vi "Magnet_PS_Main.vi"(10 "Comms Layer":T3, 11 "VISA iPS":refnum<visa-resource-name>="COM6" caption="VISA") -> (3 "Output Current (A)":dbl format="%.2g")   [LabVIEW 2019]
uses:
  Mercury iXX Modules/Public/Controls/Comms Transport Layer.ctl
  Mercury iXX Modules/Public/Libraries/Magnet/Controls/PSU Actions.ctl
  <vilib>/Instr/_visa.llb/VISA Flush IO Buffer Mask.ctl
  Magnet_PS_Global.vi
  Mercury iXX Modules/Public/Libraries/Magnet/Configuration/Set/PSU Action Status (Set).vi
  Mercury iXX Modules/Public/Libraries/Magnet/Signals/Set/Target Current (Set).vi
  Mercury iXX Modules/Mercury iXX.lvlib
  Mercury iXX Modules/Public/Libraries/Magnet.lvlib
panel:
  in  "recon_ami1700":bool
  out "lock_time_now":i32 caption="Time Elapsed"
  in  "lock_time_max":i32=600 caption="Max Time"
  in  "enable_time_limit":bool=TRUE caption="Time Limit"
  out "High BG Light?":bool
  out "current_diff":u32(colorbox) caption="Current Difference Status"
  in  "lock_unusual_manip":bool=TRUE caption="Unusual Controls"
  out "quenched_light":bool caption="Quenched"
  out "PSU_stat_hex":i32 caption="Status" format="%x"
  out "PSU_Stat":T1 caption="PSU Status"
  out "clamped_light":bool caption="Clamped"
  out "pd read":string
  out "pd_shim_2":bool
  out "pd_shim_1":bool
  in  "termination char\n(0xA = '\\n' = LF)":u8=10 format="%.0x"
  in  "VISA_ps_pd":refnum<visa-resource-name>="COM40"
  out "Status":bool
  in  "ps_ip_addr":string="192.168.24.91" caption="IP Addr."
  in  "LHe_probe_int_samp":i8=5 caption="Interval (min)"
  in  "LHe_probe_mode":enum16{"CONT", "HOLD"}(ring) caption="LHe Mode"
  in  "curr_preset":T2(ring) caption="Presets"
  in  "relay_port":u16=6722 caption="Port"
  in  "relay_address":string="192.168.24.184" caption="Addr."
  out "He Liter":dbl(slide) caption="Calibrated" scale=0.0..145.0
  out "Last Update":timestamp format="%<%Y-%m-%d %H:%M:%S>T"
  out "iPS_msg":string caption="Msg."
  out "AMI1700_status":bool caption="Status"
  in  "AMI1700_port":u16=7180 caption="Port"
  in  "AMI1700_address":string="192.168.24.134" caption="Addr."
  in  "stop":bool
  out "shim_relay_message":string caption="Msg."
  out "shim_relay_status":bool caption="Status"
  in  "Shim 2":bool caption="#2"
  in  "Shim 1":bool caption="Shim Switch Heater #1"
  in  "Save Button":bool
  in  "x":dbl=14.889566783098592 format="%#_13g"
  in  "Current NMR Central Frequency:":dbl
  in  "y":dbl=20.0
  out "SAFETY TIMEOUT":u8(slide) scale=0.0..60.0
  in  "safemode":bool
  out "Timer":dbl
  in  "Help Button":bool
  out "help_msg":string="To ramp the current above 74.8 A, or faster than 2 A/min (for I<40A), 1 A/min (for 40A<I<63A) or 0.5 A/min (for I>63A), please enter the correct password.\n\nBaseline Mode: Toggle on to ramp the magnet to 1 A below the set point for the purposes of taking a baseline. Toggle off to ramp back to the set point. If the switch heater is off, it will be turned on when this button is pressed.\n\nSafety Mode: While toggled on, switch heater will automatically turn off after 20 minutes of inactivity. Enter password to change timeout duration."
  in  "Special Functions":bool
  out "Baselinetext":string
  in  "Target Species:":dbl(ring)=42.576 items=["Proton"=42.576, "Deuteron"=6.536]
  out "Heater Status 2":u8(slide) scale=0.0..60.0
  in  "Baseline Mode":bool
  out "Heater Status":u8(slide) scale=0.0..60.0
  out "big_message":string
  in  "Set Target Frequency (MHz):":dbl max=213.8870019787944
  in  "Set Target Field (T):":dbl max=5.02365186909983 format="%#_5g"
  in  "Axis Group":string(combo)="GRPZ"
  in  "Target Current":dbl max=74.8 format="%#_5g"
  out "N2 Level":dbl(slide) scale=0.0..100.0
  out "He Level":dbl(slide) scale=0.0..45.0
  in  "all_cont_lock":bool caption="All Controls"
  out "Zerolight":bool
  out "Setlight":bool
  out "Holdlight":bool
  out "Persistent Current (A)":dbl format="%.2g"
  in  "PASSWORD:":string
  out "Heater Indicator 3":bool caption="Main Switch Heater"
  in  "Switch Heater":bool caption="Toggle"
  in  "Ramp Rate (A/min)":dbl=0.5 min=0.0 max=2.0 format="%_2f"
  out "Set Target Current (A):":cluster{dbl, dbl}(knob)={0.0, 68.56622626412835} scale=0.0..120.0 scale format="%#_5g"
  in  "To Zero":bool
  in  "To Set":bool
  in  "Hold":bool
  out "Waveform Chart":cluster{"[0]":dbl, "[1]":dbl}(graph)
  out "Output Voltage (V)":dbl format="%.3g"
  out "iPS_status":bool caption="Status"
  out "String 2":string
  # "Magnet Power Supply"
  # "/"
  # "s"
  # "For Drift Calibration:"
  # "Mercury iPS"
  # "%"
  # "L"
  # "%"
  # "Shim Relay"
  # "Known as bad."
  # "AMI1700"
  # "The ramp rate is auto-lowered when exceeding the limit that is defined in hardware as a function of output current."
  # "This toggle button changes the main & shim switch heaters together."
  # "PD Reading"
  # "Photodiodes"
  # "(hex)"
  # "Unusual Controls:\n* Press \"To Set\" or \"To Zero\" when the main+shim heaters are not all ON or OFF.\n* Change the heater status when the PS is not in \"Hold\".\n* Change the heater status when Output current != Presistent Current.\nYou might hover the mouse cursor on the \"Unusual Controls\" button\nto find the reason why controls are prohibited."
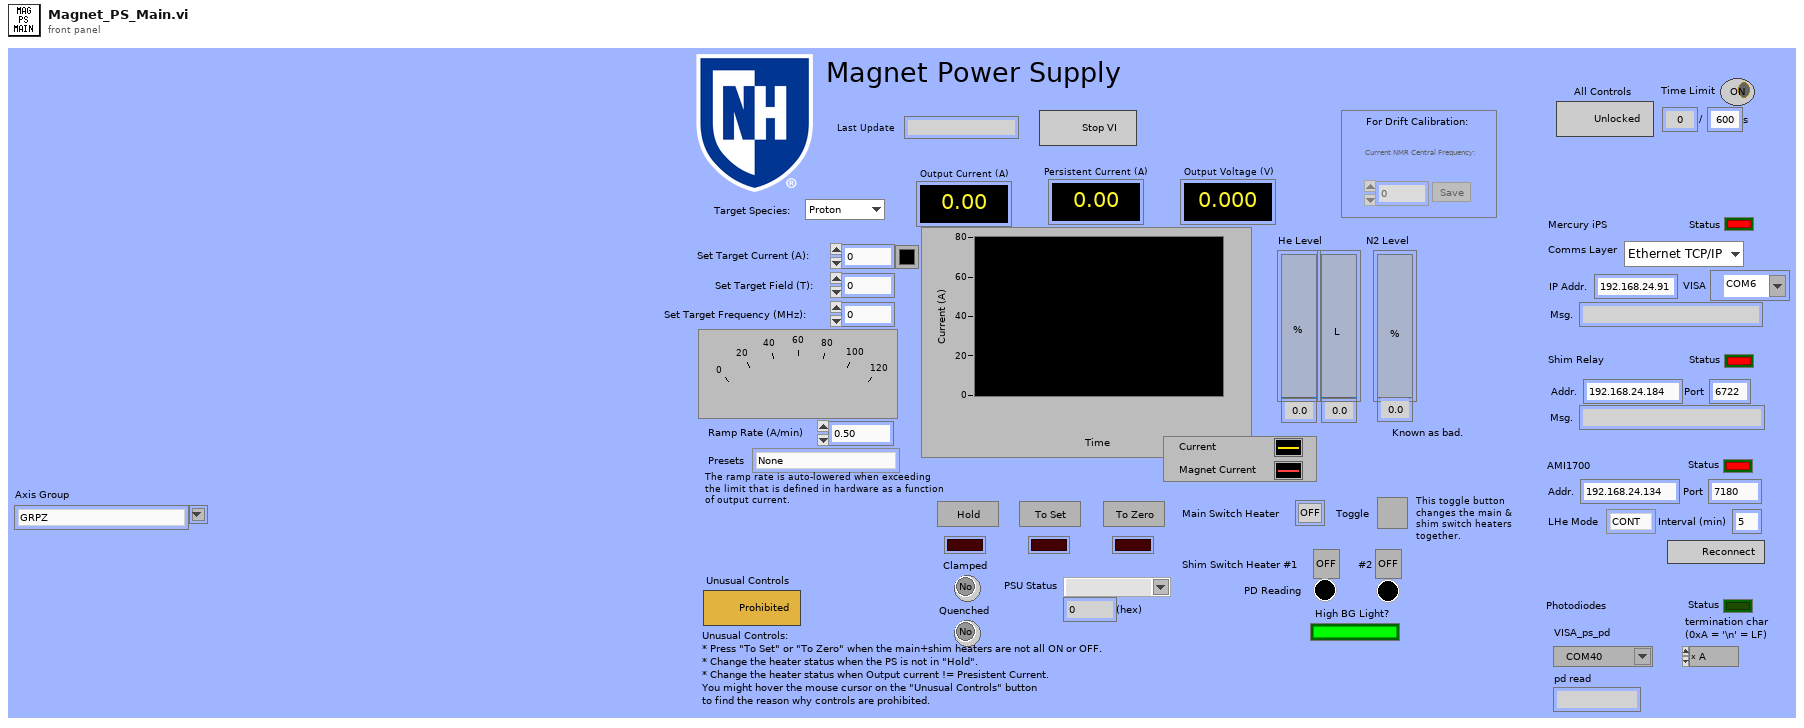
[diagram p1: front panel]
types:
  T1 = typedef "Mercury iXX.lvlib/Magnet.lvlib/PSU Actions.ctl" = string
  T2 = enum16{"None", "Up to 45 A at 2 A/m", "Up to 63 A at 1 A/m", "Up to 74.51 A at 0.5 A/m", "Up to 74.47 A at 0.5 A/m", "Down to 74 A at 0.5 A/m", "Down to 63 A at 0.5 A/m", "Down to 45 A at 1 A/m", "Down to 0 A at 2 A/m", "Down to 0 A at 0.5 A/m"}
  T3 = typedef "Mercury iXX.lvlib/Comms Transport Layer.ctl" = enum16{"Ethernet TCP/IP", "USB", "ISOBus - RS-232", "GPIB"}
  T4 = typedef "VISA Flush IO Buffer Mask.ctl" = u16
  T5 = typedef "Mercury iXX.lvlib/ISOBus Address.ctl" = i32
  T6 = typedef "Mercury iXX.lvlib/Mercury Reference.ctl" = cluster{"Comms":refnum<visa-resource-name>, "Device ID":string[], "Comms Layer":T3, "Command":string, "Query reference":T7}
  T7 = typedef "Mercury iXX.lvlib/Query Dynamic Reference.ctl" = refnum<vi>
  T8 = enum8{"Enabled", "Disabled", "Disabled and Grayed Out"}
  T9 = enum16{"None", "Up: 45 A, 2 A/m", "Up: 63 A, 1 A/m", "Up: 74.78 A, 0.5 A/m", "Down: 63 A, 0.5 A/m", "Down: 45 A, 1 A/m", "Down: 0 A, 2 A/m"}
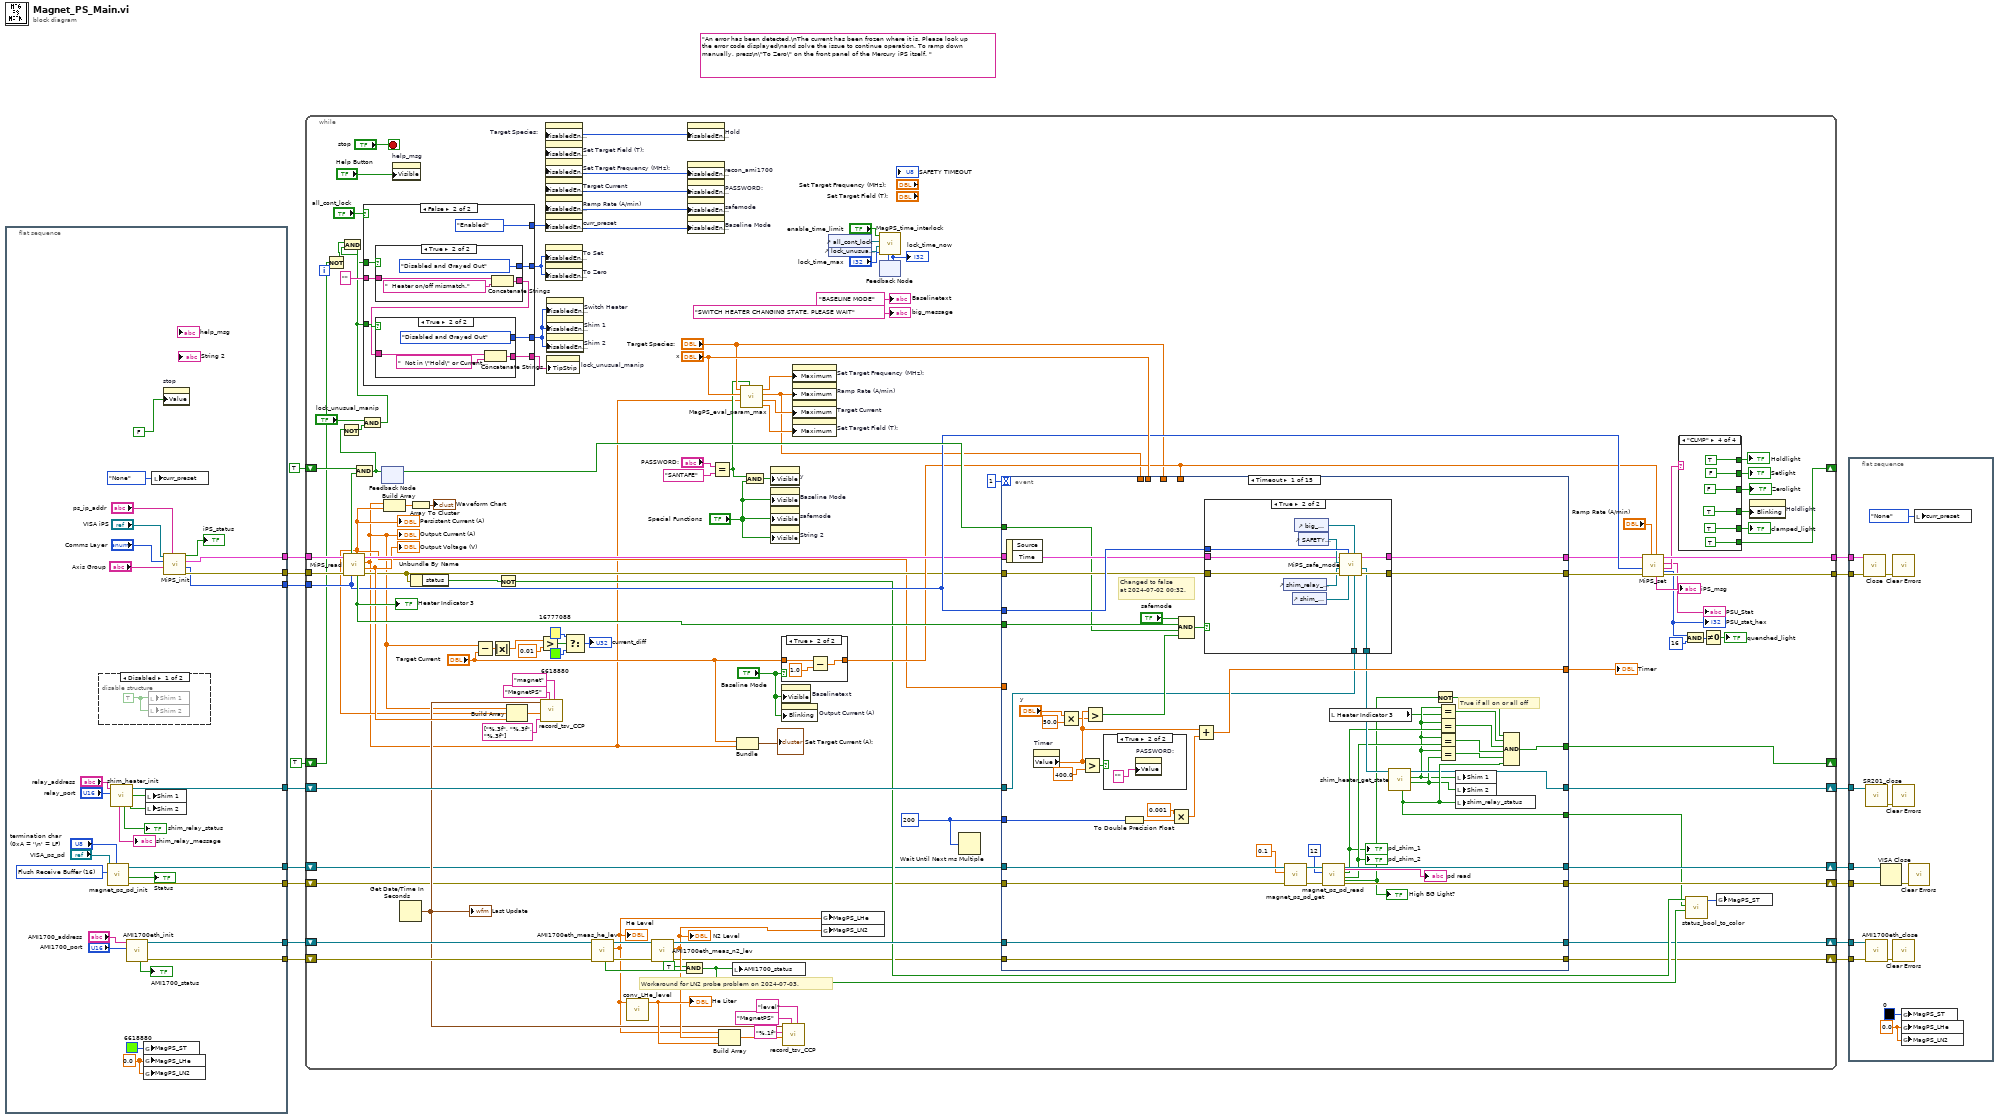
[diagram p0: block diagram]
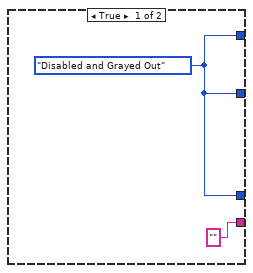
[diagram p3: hidden frame]
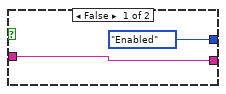
[diagram p4: hidden frame]
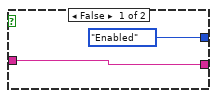
[diagram p5: hidden frame]
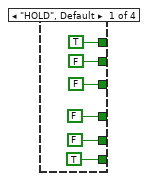
[diagram p7: hidden frame]
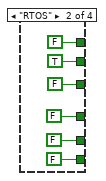
[diagram p8: hidden frame]
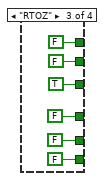
[diagram p9: hidden frame]
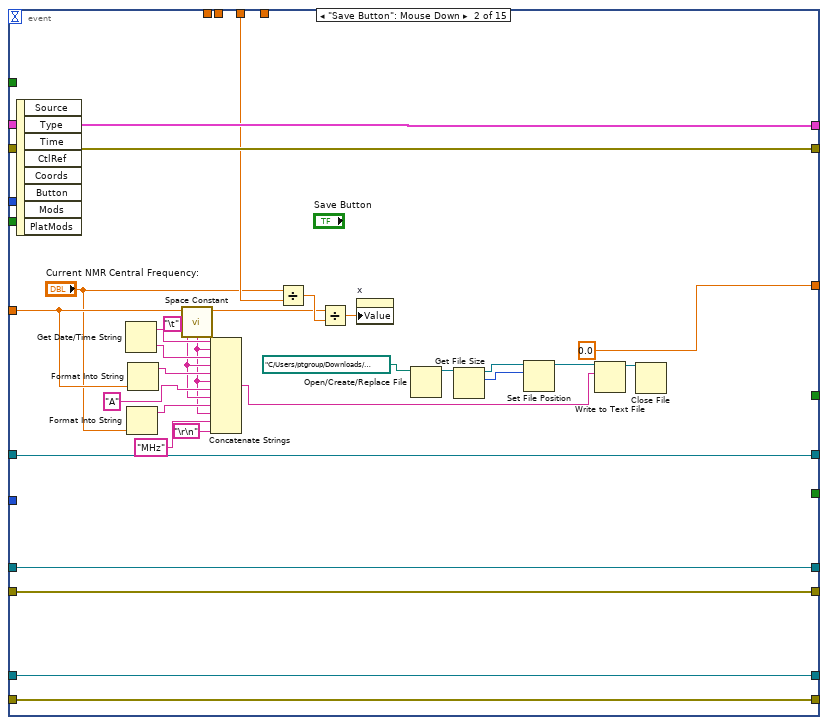
[diagram p12: hidden frame]
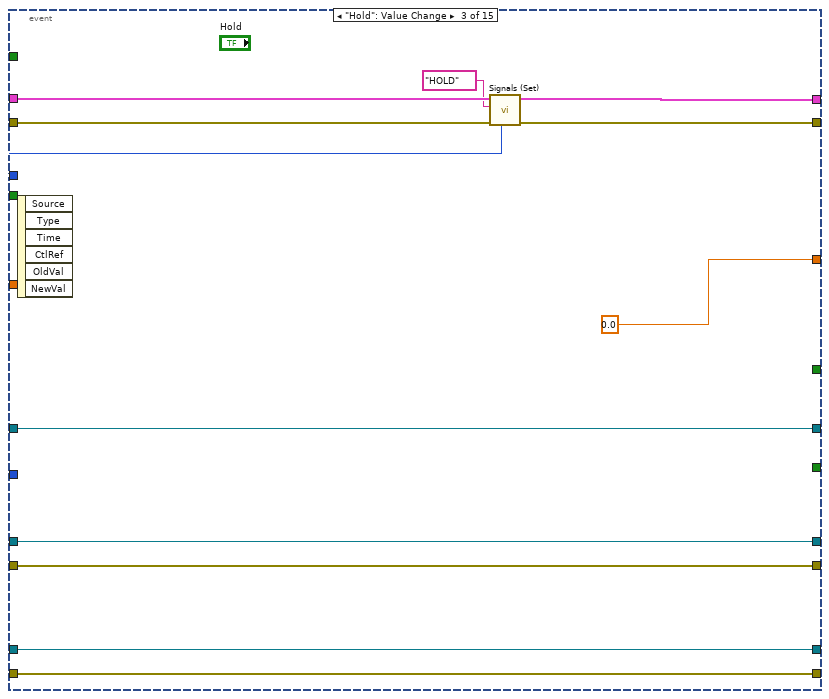
[diagram p13: hidden frame]
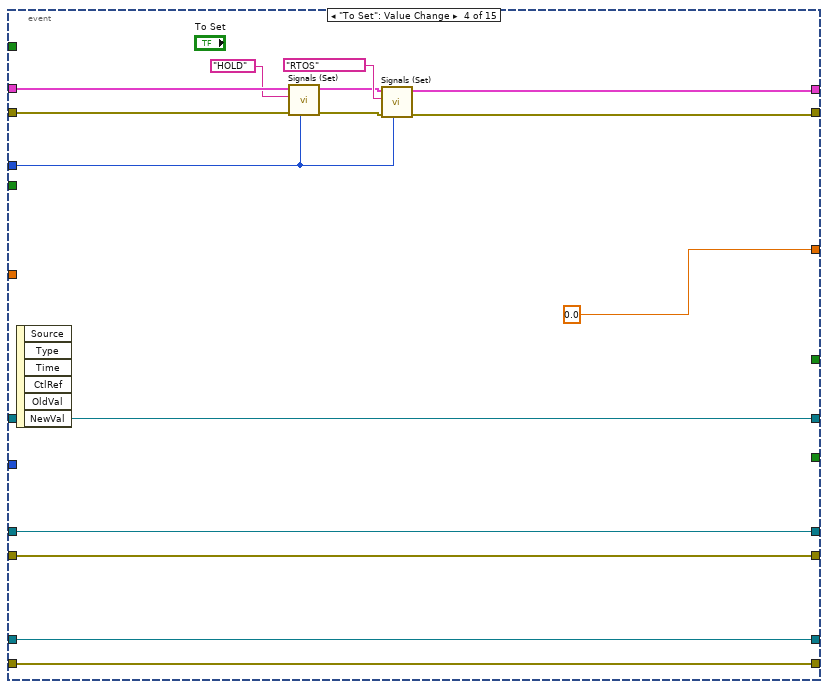
[diagram p14: hidden frame]
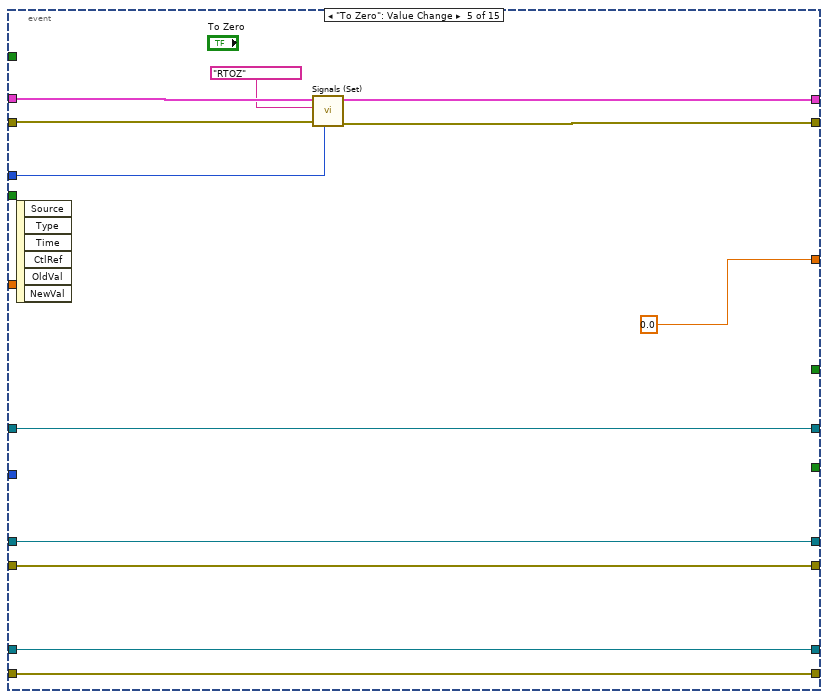
[diagram p15: hidden frame]
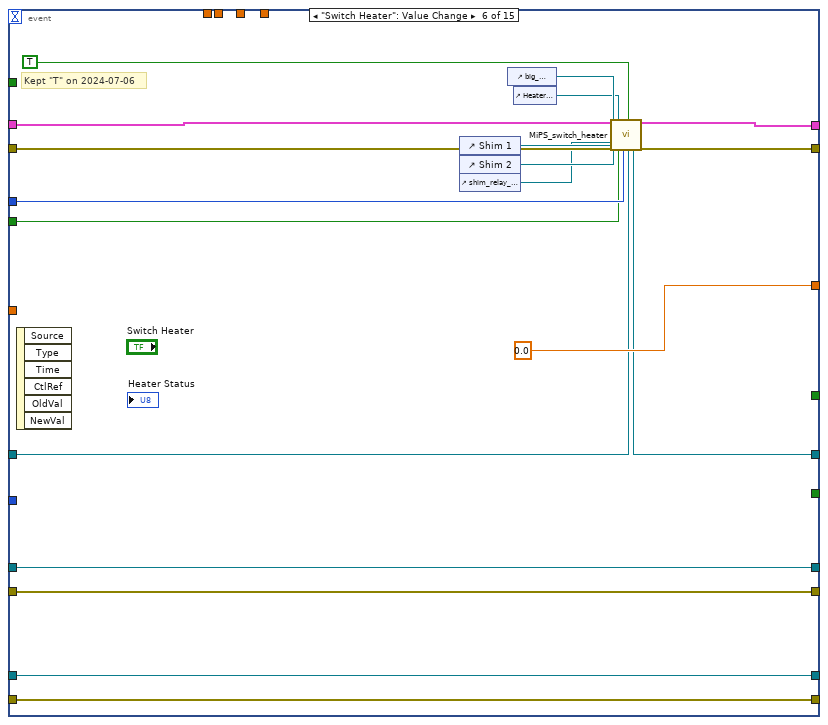
[diagram p16: hidden frame]
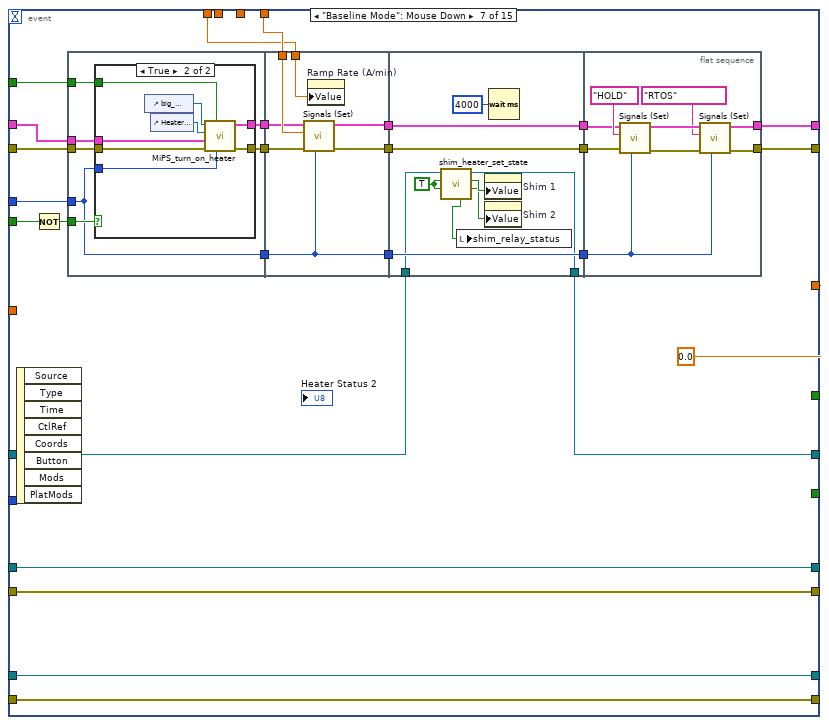
[diagram p17: hidden frame]
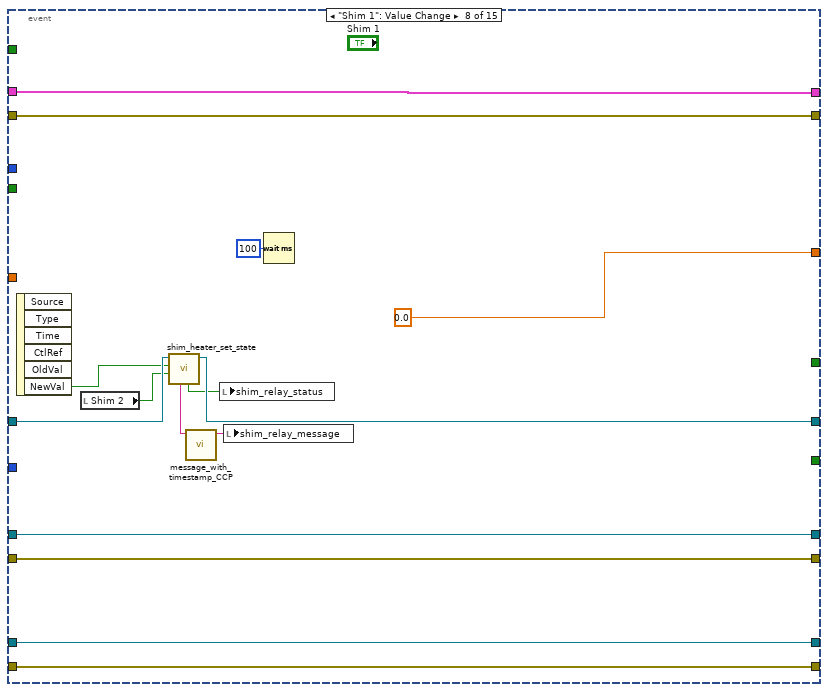
[diagram p19: hidden frame]
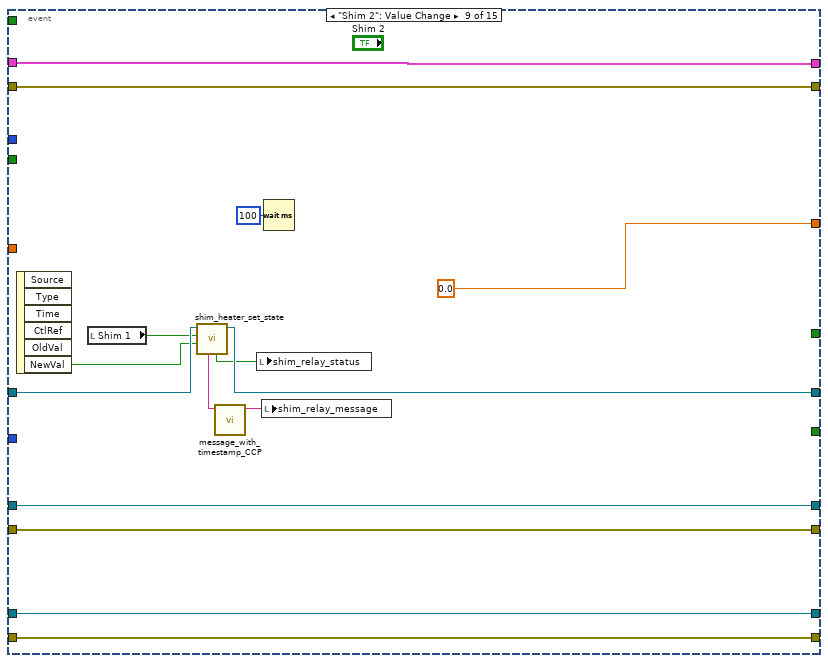
[diagram p20: hidden frame]
diagram:
  (unwired) "An error has been detected.\nThe current has been frozen where it is. Please look up the error code displayed\nand solve the issue to continue operation. To ramp down manually, press\n\"To Zero\" on the front panel of the Mercury iPS itself. " ("message")
  n1 = flat-sequence {
    tunnel: [w46] -> w17
    tunnel: [w45] -> w16
    tunnel: [w42] -> w13
    tunnel: [w37] -> w12
    tunnel: [w36] -> w11
    tunnel: [w32] -> w7
    tunnel: [w19] -> w3
    tunnel: [w21] -> w5
    frame #0 {
      w23 = T4 16 items=["Flush Receive Buffer"=16, "Write Transmit Buffer to Device"=32, "Flush Receive Buffer (No I/O)"=64, "Flush Transmit Buffer"=128] ("Mask")
      w26 = 0.0 ("MagPS_LHe")
      n2 = disable-structure shown="Disabled" {
        frame Disabled {
          w48 = TRUE ("Shim 1")
          n3 = local write "Shim 1"(w48) -> ()
          n4 = local write "Shim 2"(w48) -> ()
        }
        frame Enabled {
        }
      }
      n5 = call "magnet_ps_pd_init.vi"("termination char\n(0xA = '\\n' = LF)"="termination char\n(0xA = '\\n' = LF)", "Mask"=w23, "VISA resource name"="VISA_ps_pd") -> ("error out"=w19:errorcluster, "Status"=→"Status":bool, "VISA resource name out"=w21:refnum<visa-resource-name>)  [unwired: 6 in]
      n6 = call "shim_heater_init.vi"("port"="relay_port", "address"="relay_address") -> ("ch2"=w28:bool, "ch1"=w29:bool, "conn_id"=w32:refnum<k5>, "status"=→"shim_relay_status":bool, "message"=→"shim_relay_message":string)  [unwired: 4 in, 1 out]
      n7 = call "AMI1700eth_init.vi"("port"="AMI1700_port", "address"="AMI1700_address") -> ("error out"=w36:errorcluster, "conn_id"=w37:refnum<k5>, "status"=→"AMI1700_status":bool)  [unwired: 7 in]
      n8 = global write "Magnet_PS_Global.vi" "MagPS_ST"(u32 6618880 ("MagPS_ST")) -> ()
      n9 = global write "Magnet_PS_Global.vi" "MagPS_LHe"(w26) -> ()
      n10 = global write "Magnet_PS_Global.vi" "MagPS_LN2"(w26) -> ()
      n11 = local write "Shim 1"(w29) -> ()
      n12 = local write "Shim 2"(w28) -> ()
      n13 = local write "curr_preset"(T2."None" ("curr_preset")) -> ()
      n14 = property on="stop" class="Bool (strict)"("Value"=FALSE ("stop")) -> ()  [unwired: 2 in, 2 out]
      n15 = call "MiPS_init.vi"("ip_addr"="ps_ip_addr", "Axis Group"="Axis Group", "Comms Layer"="Comms Layer", "VISA in"="VISA iPS") -> ("error out"=w45:errorcluster, "ISOBUS address"=w42:T5, "ref_out"=w46:T6, "status"=→"iPS_status":bool)  [unwired: 4 in]
    }
  }
  n16 = while {
    tunnel: w17 -> [w156]
    tunnel: w16 -> [w157]
    tunnel: [w150] -> w15
    tunnel: [w149] -> w14
    tunnel: w13 -> [w129]
    shift-right: [w54] -> w10
    shift-left: w12 -> [w132]
    shift-right: [w55] -> w9
    shift-left: w11 -> [w134]
    shift-right: [w118] -> _
    shift-left: TRUE -> [w117]
    shift-right: [w74] -> w6
    shift-left: w7 -> [w105]
    shift-right: [w94] -> w4
    shift-left: w5 -> [w95]
    shift-right: [w92] -> w2
    shift-left: w3 -> [w93]
    shift-right: [w73] -> _
    shift-left: TRUE -> [w76]
    stop <- "stop" stop-if-true
    w137 = u32 200 ("millisecond multiple")
    # "Workaround for LN2 probe problem on 2024-07-03."
    n17 = Not(x=w76) -> (.not. x?=w50:bool)
    n18 = call "MiPS_read.vi"("ISOBUS address"=w129, "error in"=w157, "ref_in"=w156) -> ("error out"=w107:errorcluster, "Voltage"=w108:dbl, "Current"=w71:dbl, "ref_out"=w128:T6, "heater_status"=w151:bool, "Persistant Current"=w85:dbl, "current_in_range"=w127:bool)  [unwired: 2 in]
    "Output Current (A)" <- w71
    "Output Voltage (V)" <- w108
    "Heater Indicator 3" <- w151
    "Persistent Current (A)" <- w85
    n19 = And(x=w117, y=w127) -> (x .and. y?=w81:bool)
    n20 = Not(x=w81) -> (.not. x?=w82:bool)
    n21 = And(x="lock_unusual_manip", y=w82) -> (x .and. y?=w52:bool)
    n22 = And(x=w50, y=w52) -> (x .and. y?=w51:bool)
    n23 = case shown="False" "all_cont_lock" {
      tunnel: [w164 w172] -> w83
      tunnel: w52 -> [_ w167]
      tunnel: [w164 T8."Enabled" ("Disabled")] -> w53
      tunnel: [w164 w170] -> w80
      tunnel: ["" ("f") w169] -> w79
      tunnel: "" ("f") -> [_ w168]
      tunnel: w51 -> [_ w165]
      frame True {
        w164 = T8."Disabled and Grayed Out" ("Disabled")
      }
      frame False {
        n24 = case shown="True" w165 {
          tunnel: [T8."Enabled" ("Disabled") T8."Disabled and Grayed Out" ("Disabled")] -> w170
          tunnel: w168 -> [w173 w177]
          tunnel: [w173 w176] -> w166
          frame False {
          }
          frame True {
            n25 = Concatenate Strings(w177, "  Heater on/off mismatch." ("string")) -> (w176:string)
          }
        }
        n26 = case shown="True" w167 {
          tunnel: [T8."Enabled" ("Disabled") T8."Disabled and Grayed Out" ("Disabled")] -> w172
          tunnel: [w179 w183] -> w169
          tunnel: w166 -> [w179 w182]
          frame False {
          }
          frame True {
            n27 = Concatenate Strings(w182, "  Not in \"Hold\" or Current mismatch." ("msg_heater_manip")) -> (w183:string)
          }
        }
      }
    }
    n28 = feedback-in #1(w81) -> ()
    n29 = feedback #1() -> (w144:bool)  [unwired: 1 in]
    n30 = Build Array(w71, w85) -> (w148:dbl[])
    n31 = property on="help_msg" class="Str"("Visible"="Help Button") -> ()  [unwired: 2 in, 2 out]
    n32 = Get Date/Time In Seconds() -> (seconds since 1Jan1904=w98:timestamp)
    "Last Update" <- w98
    n33 = Array To Cluster(array=w148) -> (cluster=→"Waveform Chart":cluster{"[0]":dbl, "[1]":dbl})
    n34 = Unbundle By Name(w107) -> ("status"=w106:bool)
    n35 = Subtract(x=w71, y="Target Current") -> (x-y=w70:dbl)
    n36 = Absolute Value(x=w70) -> (abs(x)=w68:dbl)
    n37 = Not(x=w106) -> (.not. x?=w103:bool)
    n38 = Build Array(w71, w85, w108) -> (w110:dbl[])
    n39 = Greater?(x=w68, y=0.01) -> (0:w67:bool)
    n40 = call "record_tsv_CCP.vi"("file_name"="magnet", "folder_name"="MagnetPS", "format_array"=string[] ["%.3f", "%.3f", "%.3f"], "value_array"=w110, "time"=w98) -> ()  [unwired: 5 in, 2 out]
    n41 = property on="Target Species:" class="Ring (strict)"("DisabledEnum"=w53) -> ()  [unwired: 2 in, 2 out]
    n42 = property on="Set Target Field (T):" class="DigNum (strict)"("DisabledEnum"=w53) -> ()  [unwired: 2 in, 2 out]
    n43 = property on="Set Target Frequency (MHz):" class="DigNum (strict)"("DisabledEnum"=w53) -> ()  [unwired: 2 in, 2 out]
    n44 = property on="Target Current" class="DigNum (strict)"("DisabledEnum"=w53) -> ()  [unwired: 2 in, 2 out]
    n45 = property on="Ramp Rate (A/min)" class="DigNum (strict)"("DisabledEnum"=w53) -> ()  [unwired: 2 in, 2 out]
    n46 = property on="curr_preset" class="Enum (strict)"("DisabledEnum"=w53) -> ()  [unwired: 2 in, 2 out]
    n47 = property on="To Set" class="Bool"("DisabledEnum"=w80) -> ()  [unwired: 2 in, 2 out]
    n48 = property on="To Zero" class="Bool"("DisabledEnum"=w80) -> ()  [unwired: 2 in, 2 out]
    n49 = property on="Switch Heater" class="Bool"("DisabledEnum"=w83) -> ()  [unwired: 2 in, 2 out]
    n50 = property on="Shim 1" class="Bool (strict)"("DisabledEnum"=w83) -> ()  [unwired: 2 in, 2 out]
    n51 = property on="Shim 2" class="Bool (strict)"("DisabledEnum"=w83) -> ()  [unwired: 2 in, 2 out]
    n52 = property on="lock_unusual_manip" class="Bool (strict)"("TipStrip"=w79) -> ()  [unwired: 2 in, 2 out]
    n53 = Select(t=u32 16777088 ("THCD401_ST"), s=w67, f=u32 6618880 ("THCD401_ST")) -> (s? t:f=→"current_diff":u32)
    n54 = call "AMI1700eth_meas_he_lev.vi"("error in"=w134, "conn_id_in"=w132) -> ("error out"=w133:errorcluster, "level"=w96:dbl, "conn_id_out"=w131:refnum<k5>, "status"=w130:bool)  [unwired: 5 in, 1 out]
    "He Level" <- w96
    n55 = call "conv_LHe_level.vi"("level_in"=w96) -> ("level_out"=w113:dbl)  [unwired: 10 in]
    "He Liter" <- w113
    n56 = call "AMI1700eth_meas_n2_lev.vi"("error in"=w133, "conn_id_in"=w131) -> ("error out"=w56:errorcluster, "level"=w100:dbl, "conn_id_out"=w104:refnum<k5>)  [unwired: 6 in, 1 out]
    "N2 Level" <- w100
    n57 = And(x=TRUE, y=w130) -> (x .and. y?=w101:bool)
    n58 = property on="Hold" class="Bool"("DisabledEnum"=w53) -> ()  [unwired: 2 in, 2 out]
    n59 = property on="recon_ami1700" class="Bool"("DisabledEnum"=w53) -> ()  [unwired: 2 in, 2 out]
    n60 = property on="PASSWORD:" class="Str"("DisabledEnum"=w53) -> ()  [unwired: 2 in, 2 out]
    n61 = property on="safemode" class="Bool (strict)"("DisabledEnum"=w53) -> ()  [unwired: 2 in, 2 out]
    n62 = property on="Baseline Mode" class="Bool (strict)"("DisabledEnum"=w53) -> ()  [unwired: 2 in, 2 out]
    n63 = Equal?(x="PASSWORD:", y="SANTAFE") -> (x = y?=w121:bool)
    n64 = Build Array(w96, w100, w113) -> (w114:dbl[])
    n65 = local write "AMI1700_status"(w101) -> ()
    n66 = Bundle("Target Current"="Target Current", "Current"=w71) -> (→"Set Target Current (A):":cluster{"Target Current":dbl, "Current":dbl})  [unwired: 1 in]
    n67 = call "MagPS_eval_param_max.vi"("admin_mode"=w121, "Current"=w71, "x"="x", "Target Species"="Target Species:") -> ("target_field_max"=w120:dbl, "target_current_max"=w145:dbl, "ramp_rate_max"=w119:dbl, "target_frequency_max"=w141:dbl)  [unwired: 4 in]
    n68 = And(x=w121, y="Special Functions") -> (x .and. y?=w136:bool)
    n69 = property on="y" class="DigNum (strict)"("Visible"=w136) -> ()  [unwired: 2 in, 2 out]
    n70 = property on="Baseline Mode" class="Bool (strict)"("Visible"="Special Functions") -> ()  [unwired: 2 in, 2 out]
    n71 = property on="safemode" class="Bool (strict)"("Visible"="Special Functions") -> ()  [unwired: 2 in, 2 out]
    n72 = property on="String 2" class="Str"("Visible"="Special Functions") -> ()  [unwired: 2 in, 2 out]
    n73 = case shown="True" "Baseline Mode" {
      tunnel: "Target Current" -> [w185 w187]
      tunnel: [w185 w186] -> w124
      frame False {
      }
      frame True {
        n74 = Subtract(x=w187, y=1.0) -> (x-y=w186:dbl)
      }
    }
    n75 = property on="Baselinetext" class="Str"("Visible"="Baseline Mode") -> ()  [unwired: 2 in, 2 out]
    n76 = property on="Output Current (A)" class="DigNum (strict)"("Blinking"="Baseline Mode") -> ()  [unwired: 2 in, 2 out]
    n77 = call "record_tsv_CCP.vi"("file_name"="level", "folder_name"="MagnetPS", "value_array"=w114, "format"="%.1f", "time"=w98) -> ()  [unwired: 5 in, 2 out]
    n78 = property on="Set Target Frequency (MHz):" class="DigNum (strict)"("Maximum"=w141) -> ()  [unwired: 2 in, 2 out]
    n79 = property on="Ramp Rate (A/min)" class="DigNum (strict)"("Maximum"=w119) -> ()  [unwired: 2 in, 2 out]
    n80 = property on="Target Current" class="DigNum (strict)"("Maximum"=w145) -> ()  [unwired: 2 in, 2 out]
    n81 = property on="Set Target Field (T):" class="DigNum (strict)"("Maximum"=w120) -> ()  [unwired: 2 in, 2 out]
    n82 = global write "Magnet_PS_Global.vi" "MagPS_LHe"(w96) -> ()
    n83 = global write "Magnet_PS_Global.vi" "MagPS_LN2"(w100) -> ()
    n84 = control-ref of="all_cont_lock"() -> (w62:refnum<vi>)
    n85 = control-ref of="lock_unusual_manip"() -> (w57:refnum<vi>)
    n86 = feedback #2() -> (w59:i32)  [unwired: 1 in]
    n87 = call "MagPS_time_interlock.vi"("time_in"=w59, "time_max"="lock_time_max", "unusual_cont_lock"=w57, "all_cont_lock"=w62, "enable_time_limit"="enable_time_limit") -> ("time_out"=w60:i32)  [unwired: 5 in, 1 out]
    "lock_time_now" <- w60
    n88 = feedback-in #2(w60) -> ()
    n89 = Wait Until Next ms Multiple(millisecond multiple=w137) -> ()  [unwired: 1 out]
    n90 = event shown="[0] Timeout" {
      selector: _ -> [_ _ _ _ _ _ _ _ _ _ _ _ _ _ _]
      dyn-events: _ -> [_ _ _ _ _ _ _ _ _ _ _ _ _ _ _]
      timeout: 1 -> [_ _ _ _ _ _ _ _ _ _ _ _ _ _ _]
      tunnel: [w250 w303 w315 w331 w342 w361 w382 w445 w460 w474 w482 w495 w511 w541 w547] -> w125
      tunnel: w128 -> [w251 w303 w316 w330 w343 w362 w386 w445 w460 w474 w482 w495 w511 w541 w547]
      tunnel: w151 -> [w243 _ _ _ _ w345 w388 _ _ _ _ _ _ _ _]
      tunnel: w107 -> [w252 w304 w314 w329 w341 w360 w384 w444 w459 w473 w481 w494 w510 w540 w546]
      tunnel: [w249 w304 w313 w328 w340 w359 w383 w444 w459 w473 w481 w494 w510 w540 w546] -> w160
      tunnel: w144 -> [w242 _ _ _ _ _ w385 _ _ _ _ _ _ _ _]
      tunnel: w129 -> [w253 _ w312 w327 w339 w358 w381 _ _ _ _ _ _ _ _]
      tunnel: "x" -> [_ _ _ _ _ _ _ _ _ w471 w487 w497 _ _ _]
      tunnel: "Target Species:" -> [_ w301 _ _ _ _ _ _ _ w469 w485 w499 _ _ _]
      tunnel: w124 -> [_ _ _ _ _ _ w376 _ _ _ _ _ _ _ _]
      tunnel: [w256 0.0 0.0 0.0 0.0 0.0 0.0 0.0 0.0 0.0 0.0 0.0 w509 w538 0.0 ("Timer")] -> w138
      tunnel: w137 -> [w260 _ _ _ _ _ _ _ _ _ _ _ _ _ _]
      tunnel: w85 -> [_ w290 _ _ _ _ _ _ _ _ _ _ w509 _ _]
      tunnel: w119 -> [_ _ _ _ _ _ w375 _ _ _ _ _ _ _ _]
      tunnel: w105 -> [w239 w280 w310 w323 w337 w356 w368 w442 w457 w466 w479 w492 w508 w539 w548]
      tunnel: [w227 w280 w310 w323 w337 w355 w367 w441 w456 w466 w479 w492 w508 w539 w548] -> w74
      tunnel: w104 -> [w214 w277 w306 w318 w333 w347 w364 w433 w448 w463 w476 w489 w502 w542 w558]
      tunnel: w95 -> [w237 w279 w309 w324 w335 w354 w366 w435 w449 w465 w478 w491 w504 w537 w550]
      tunnel: [w238 w279 w309 w324 w335 w354 w366 w435 w449 w465 w478 w491 w504 w537 w550] -> w94
      tunnel: w93 -> [w234 w278 w308 w325 w336 w353 w365 w434 w450 w464 w477 w490 w503 w536 w549]
      tunnel: [w232 w278 w308 w325 w336 w353 w365 w434 w450 w464 w477 w490 w503 w536 w549] -> w92
      tunnel: [w229 _ _ _ _ _ _ _ _ _ _ _ _ _ _] -> w75
      tunnel: [w226 _ _ _ _ _ _ _ _ _ _ _ _ _ _] -> w73
      tunnel: [w214 w277 w306 w318 w333 w347 w364 w433 w448 w463 w476 w489 w502 w535 w553] -> w54
      tunnel: [w213 w276 w305 w317 w332 w346 w363 w432 w447 w462 w475 w488 w501 w534 w552] -> w55
      tunnel: w56 -> [w213 w276 w305 w317 w332 w346 w363 w432 w447 w462 w475 w488 w501 w533 w551]
      event Timeout {
        # "Changed to false\nat 2024-07-02 00:32."
        # "True if all on or all off"
        n91 = event-data() -> ()  [unwired: 1 in, 2 out]
        n92 = property on="Timer" class="DigNum (strict)"() -> ("Value"=w248:dbl)  [unwired: 2 in, 2 out]
        n93 = Multiply(x="y", y=50.0) -> (x*y=w245:dbl)
        n94 = Greater?(x=w248, y=400.0) -> (0:w254:bool)
        n95 = Greater?(x=w248, y=w245) -> (0:w241:bool)
        n96 = case shown="True" w254 {
          frame False {
          }
          frame True {
            n97 = property on="PASSWORD:" class="Str"("Value"="" ("PASSWORD:")) -> ()  [unwired: 2 in, 2 out]
          }
        }
        n98 = To Double Precision Float(number=w260) -> (double precision float=w259:dbl)
        n99 = Multiply(x=0.001, y=w259) -> (x*y=w257:dbl)
        n100 = Compound Arithmetic op=AND("safemode", w243, w242, w241) -> (w244:bool)
        n101 = Add(x=w248, y=w257) -> (x+y=w256:dbl)
        n102 = case shown="True" w244 {
          tunnel: w251 -> [w263 w266]
          tunnel: [w263 w274] -> w250
          tunnel: w252 -> [w262 w273]
          tunnel: [w262 w272] -> w249
          tunnel: w253 -> [_ w271]
          tunnel: w239 -> [w261 w265]
          tunnel: [w261 w264] -> w228
          frame False {
          }
          frame True {
            n103 = control-ref of="shim_relay_status"() -> (w269:refnum<vi>)
            n104 = control-ref of="shim_relay_message"() -> (w268:refnum<vi>)
            n105 = control-ref of="big_message"() -> (w267:refnum<vi>)
            n106 = control-ref of="SAFETY TIMEOUT"() -> (w270:refnum<vi>)
            n107 = call "MiPS_safe_mode.vi"("conn_id_in"=w265, "ref_big_msg"=w267, "ref_relay_msg"=w268, "ISOBUS address"=w271, "error in"=w273, "ref_relay_status"=w269, "ref_timeout_slider"=w270, "ref_in"=w266) -> ("error out"=w272:errorcluster, "conn_id_out"=w264:refnum<k5>, "ref_out"=w274:T6)  [unwired: 1 in]
          }
        }
        n108 = call "magnet_ps_pd_get.vi"("error in (no error)"=w234, "Wait untill read (S)"=0.1, "VISA resource name"=w237) -> ("error out"=w233:errorcluster, "VISA resource name out"=w236:refnum<visa-resource-name>)  [unwired: 7 in]
        n109 = call "magnet_ps_pd_read.vi"("error in (no error)"=w233, "byte count to read"=u32 12, "VISA resource name"=w236) -> ("error out"=w232:errorcluster, "Shim Coil 2"=w223:bool, "Shim Coil 1"=w222:bool, "VISA resource name out"=w238:refnum<visa-resource-name>, "read buffer"=→"pd read":string, "High Background?"=w217:bool)  [unwired: 2 in, 1 out]
        "pd_shim_1" <- w222
        "pd_shim_2" <- w223
        "High BG Light?" <- w217
        n110 = local read "Heater Indicator 3"() -> (w218:bool)
        n111 = call "shim_heater_get_state.vi"("conn_id_in"=w228) -> ("ch2"=w225:bool, "ch1"=w219:bool, "conn_id_out"=w227:refnum<k5>, "status"=w229:bool)  [unwired: 6 in, 1 out]
        n112 = Not(x=w217) -> (.not. x?=w215:bool)
        n113 = Equal?(x=w219, y=w218) -> (x = y?=w216:bool)
        n114 = Equal?(x=w219, y=w222) -> (x = y?=w220:bool)
        n115 = Equal?(x=w219, y=w223) -> (x = y?=w221:bool)
        n116 = Equal?(x=w219, y=w225) -> (x = y?=w224:bool)
        n117 = local write "Shim 1"(w219) -> ()
        n118 = local write "Shim 2"(w225) -> ()
        n119 = local write "shim_relay_status"(w229) -> ()
        n120 = Compound Arithmetic op=AND(w215, w216, w220, w221, w224, w229) -> (w226:bool)
      }
      event "Save Button": Mouse Down {
        w287 = "\t"
        n121 = event-data() -> ()  [unwired: 1 in, 8 out]
        n122 = Get Date/Time String() -> (date string=w292:string, time string=w291:string)  [unwired: 3 in]
        n123 = Format Into String("Current NMR Central Frequency:") -> (resulting string=w285:string)  [unwired: 3 in, 1 out]
        n124 = Format Into String(w290) -> (resulting string=w289:string)  [unwired: 3 in, 1 out]
        n125 = call <vilib>:"Space Constant.vi"() -> ("String"=w284:string)
        n126 = Concatenate Strings(w292, w284, w291, w287, w289, w284, "A", w287, w285, w284, "MHz", "\r\n") -> (w281:string)
        n127 = Divide(x="Current NMR Central Frequency:", y=w301) -> (x/y=w300:dbl)
        n128 = Divide(x=w290, y=w300) -> (x/y=w299:dbl)
        n129 = property on="x" class="DigNum (strict)"("Value"=w299) -> ()  [unwired: 2 in, 2 out]
        n130 = Open/Create/Replace File(file path (use dialog)=path "C:/Users/ptgroup/Downloads/ipsControl2013 new Folder/ipsControl2013 new Folder/C/Users/poltarg/Documents/currentcal.txt" ("file (use dialog)")) -> (refnum out=w297:refnum<file>)  [unwired: 5 in, 2 out]
        n131 = Get File Size(file=w297) -> (refnum out=w296:refnum<file>, size (in bytes)=w295:i64)  [unwired: 1 in, 1 out]
        n132 = Set File Position(offset (in bytes) (0)=w295, refnum=w296) -> (refnum out=w294:refnum<file>)  [unwired: 2 in, 1 out]
        n133 = Write to Text File(file (use dialog)=w294, text=w281) -> (refnum out=w293:refnum<file>)  [unwired: 2 in, 2 out]
        n134 = Close File(refnum=w293) -> ()  [unwired: 1 in, 2 out]
      }
      event "Hold": Value Change {
        n135 = event-data() -> ()  [unwired: 1 in, 6 out]
        n136 = call-poly "Signals (Set).vi"("ISOBUS address"=w312, "error in"=w314, "PSU Act Stat"=T1 "HOLD", "Mercury Reference In"=w316) -> ("error out"=w313:errorcluster, "Mercury Reference Out"=w315:T6)  [unwired: 4 in, 2 out]
      }
      event "To Set": Value Change {
        n137 = event-data() -> ()  [unwired: 1 in, 6 out]
        n138 = call-poly "Signals (Set).vi"("ISOBUS address"=w327, "error in"=w329, "PSU Act Stat"=T1 "HOLD", "Mercury Reference In"=w330) -> ("error out"=w319:errorcluster, "Mercury Reference Out"=w320:T6)  [unwired: 4 in, 2 out]
        n139 = call-poly "Signals (Set).vi"("ISOBUS address"=w327, "error in"=w319, "PSU Act Stat"=T1 "RTOS", "Mercury Reference In"=w320) -> ("error out"=w328:errorcluster, "Mercury Reference Out"=w331:T6)  [unwired: 4 in, 2 out]
      }
      event "To Zero": Value Change {
        n140 = event-data() -> ()  [unwired: 1 in, 6 out]
        n141 = call-poly "Signals (Set).vi"("ISOBUS address"=w339, "error in"=w341, "PSU Act Stat"=T1 "RTOZ", "Mercury Reference In"=w343) -> ("error out"=w340:errorcluster, "Mercury Reference Out"=w342:T6)  [unwired: 4 in, 2 out]
      }
      event "Switch Heater": Value Change {
        # "Kept \"T\" on 2024-07-06"
        n142 = event-data() -> ()  [unwired: 1 in, 6 out]
        n143 = control-ref of="Shim 1"() -> (w350:refnum<vi>)
        n144 = control-ref of="Shim 2"() -> (w349:refnum<vi>)
        n145 = control-ref of="shim_relay_status"() -> (w348:refnum<vi>)
        n146 = control-ref of="big_message"() -> (w352:refnum<vi>)
        n147 = control-ref of="Heater Status"() -> (w351:refnum<vi>)
        n148 = call "MiPS_switch_heater.vi"("ref_big_msg"=w352, "ref_shim_relay_ch1"=w350, "ref_shim_relay_ch2"=w349, "ref_shim_relay_status"=w348, "error in"=w360, "ref_timeout_slider"=w351, "heater_status_now"=w345, "ref_in"=w362, "ISOBUS address"=w358, "switching_allowed"=TRUE, "conn_id_in"=w356) -> ("conn_id_out"=w355:refnum<k5>, "ref_out"=w361:T6, "error out"=w359:errorcluster)  [unwired: 6 in]
      }
      event "Baseline Mode": Mouse Down {
        n149 = event-data() -> ()  [unwired: 1 in, 8 out]
        n150 = Not(x=w388) -> (.not. x?=w387:bool)
        n151 = flat-sequence {
          tunnel: w387 -> [w395]
          tunnel: w386 -> [w394]
          tunnel: w385 -> [w393]
          tunnel: w384 -> [w392]
          tunnel: [w391] -> w379
          tunnel: [w390] -> w378
          tunnel: w381 -> [w389]
          tunnel: [w389] -> w377
          tunnel: w379 -> [w409]
          tunnel: w378 -> [w410]
          tunnel: [w408] -> w374
          tunnel: w377 -> [w411]
          tunnel: [w411] -> w372
          tunnel: w376 -> [w412]
          tunnel: [w407] -> w370
          tunnel: w375 -> [w406]
          tunnel: w374 -> [w422]
          tunnel: [w422] -> w373
          tunnel: w372 -> [w421]
          tunnel: [w421] -> w371
          tunnel: w370 -> [w420]
          tunnel: [w420] -> w369
          tunnel: w368 -> [w418]
          tunnel: [w416] -> w367
          tunnel: [w430] -> w382
          tunnel: [w428] -> w383
          tunnel: w373 -> [w424]
          tunnel: w371 -> [w425]
          tunnel: w369 -> [w423]
          frame #0 {
            n152 = case shown="True" w395 {
              tunnel: w394 -> [w396 w405]
              tunnel: w393 -> [_ w404]
              tunnel: w392 -> [w397 w403]
              tunnel: [w397 w402] -> w391
              tunnel: [w396 w401] -> w390
              tunnel: w389 -> [_ w400]
              frame False {
              }
              frame True {
                n153 = control-ref of="big_message"() -> (w398:refnum<vi>)
                n154 = control-ref of="Heater Status 2"() -> (w399:refnum<vi>)
                n155 = call "MiPS_turn_on_heater.vi"("ISOBUS address"=w400, "switching_allowed"=w404, "error in"=w403, "ref_in"=w405, "ref_slider"=w399, "ref_big_msg"=w398) -> ("error out"=w402:errorcluster, "ref_out"=w401:T6)  [unwired: 4 in]
              }
            }
          }
          frame #1 {
            n156 = call-poly "Signals (Set).vi"("ISOBUS address"=w411, "error in"=w409, "Target Current"=w412, "Mercury Reference In"=w410) -> ("error out"=w407:errorcluster, "Mercury Reference Out"=w408:T6)  [unwired: 4 in, 2 out]
            n157 = property on="Ramp Rate (A/min)" class="DigNum (strict)"("Value"=w406) -> ()  [unwired: 2 in, 2 out]
          }
          frame #2 {
            w417 = TRUE
            n158 = call "shim_heater_set_state.vi"("state_ch2"=w417, "state_ch1"=w417, "conn_id_in"=w418) -> ("ch2"=w414:bool, "ch1"=w415:bool, "conn_id_out"=w416:refnum<k5>, "status"=w413:bool)  [unwired: 3 in, 2 out]
            n159 = local write "shim_relay_status"(w413) -> ()
            n160 = property on="Shim 1" class="Bool (strict)"("Value"=w415) -> ()  [unwired: 2 in, 2 out]
            n161 = property on="Shim 2" class="Bool (strict)"("Value"=w414) -> ()  [unwired: 2 in, 2 out]
            n162 = Wait (ms)(milliseconds to wait=u32 4000) -> ()  [unwired: 1 out]
          }
          frame #3 {
            n163 = call-poly "Signals (Set).vi"("ISOBUS address"=w425, "error in"=w423, "PSU Act Stat"=T1 "HOLD", "Mercury Reference In"=w424) -> ("error out"=w429:errorcluster, "Mercury Reference Out"=w431:T6)  [unwired: 4 in, 2 out]
            n164 = call-poly "Signals (Set).vi"("ISOBUS address"=w425, "error in"=w429, "PSU Act Stat"=T1 "RTOS", "Mercury Reference In"=w431) -> ("error out"=w428:errorcluster, "Mercury Reference Out"=w430:T6)  [unwired: 4 in, 2 out]
          }
        }
      }
      event "Shim 1": Value Change {
        n165 = event-data() -> ("NewVal"=w440:bool)  [unwired: 1 in, 5 out]
        n166 = local read "Shim 2"() -> (w439:bool)
        n167 = call "shim_heater_set_state.vi"("state_ch2"=w439, "state_ch1"=w440, "conn_id_in"=w442) -> ("conn_id_out"=w441:refnum<k5>, "status"=w437:bool, "message"=w438:string)  [unwired: 3 in, 3 out]
        n168 = call "message_with_timestamp_CCP.vi"("message_in"=w438) -> ("message_out"=w443:string)  [unwired: 10 in]
        n169 = local write "shim_relay_status"(w437) -> ()
        n170 = local write "shim_relay_message"(w443) -> ()
        n171 = Wait (ms)(milliseconds to wait=u32 100) -> ()  [unwired: 1 out]
      }
      event "Shim 2": Value Change {
        n172 = event-data() -> ("NewVal"=w454:bool)  [unwired: 1 in, 5 out]
        n173 = local read "Shim 1"() -> (w455:bool)
        n174 = call "shim_heater_set_state.vi"("state_ch2"=w454, "state_ch1"=w455, "conn_id_in"=w457) -> ("conn_id_out"=w456:refnum<k5>, "status"=w452:bool, "message"=w453:string)  [unwired: 3 in, 3 out]
        n175 = call "message_with_timestamp_CCP.vi"("message_in"=w453) -> ("message_out"=w458:string)  [unwired: 10 in]
        n176 = local write "shim_relay_status"(w452) -> ()
        n177 = local write "shim_relay_message"(w458) -> ()
        n178 = Wait (ms)(milliseconds to wait=u32 100) -> ()  [unwired: 1 out]
      }
      event "Target Current": Value Change {
        n179 = event-data() -> ("NewVal"=w472:dbl)  [unwired: 1 in]
        n180 = Divide(x=w472, y=w471) -> (x/y=w470:dbl)
        n181 = local write "Set Target Field (T):"(w470) -> ()
        n182 = Multiply(x=w470, y=w469) -> (x*y=w468:dbl)
        n183 = local write "Set Target Frequency (MHz):"(w468) -> ()
      }
      event "Set Target Field (T):": Value Change {
        n184 = event-data() -> ("NewVal"=w484:dbl)  [unwired: 1 in]
        n185 = Multiply(x=w485, y=w484) -> (x*y=w483:dbl)
        n186 = Multiply(x=w487, y=w484) -> (x*y=w486:dbl)
        n187 = local write "Set Target Frequency (MHz):"(w483) -> ()
        n188 = local write "Target Current"(w486) -> ()
      }
      event "Set Target Frequency (MHz):": Value Change {
        n189 = event-data() -> ("NewVal"=w500:dbl)  [unwired: 1 in]
        n190 = Divide(x=w500, y=w499) -> (x/y=w498:dbl)
        n191 = Multiply(x=w497, y=w498) -> (x*y=w496:dbl)
        n192 = local write "Set Target Field (T):"(w498) -> ()
        n193 = local write "Target Current"(w496) -> ()
      }
      event "curr_preset": Value Change {
        n194 = event-data() -> ("NewVal"=w505:T2)  [unwired: 1 in, 5 out]
        n195 = Not Equal?(x=T9."None" ("NewVal"), y=w505) -> (x != y?=w506:bool)
        n196 = case shown="True" w506 {
          tunnel: w505 -> [_ w513]
          frame False {
          }
          frame True {
            n197 = case shown="\"Up to 74.47 A at 0.5 A/m\"" w513 {
              tunnel: [45.0 ("Target Current") 63.0 ("Target Current") 74.51 ("Target Current") 74.47 ("Target Current") 74.0 ("Target Current") 63.0 ("Target Current") 45.0 ("Target Current") 0.0 ("Target Current") 0.0 ("Target Current")] -> w512
              tunnel: [2.0 ("Ramp Rate (A/min)") 1.0 ("Ramp Rate (A/min)") 0.5 ("Ramp Rate (A/min)") 0.5 ("Ramp Rate (A/min)") 0.5 ("Ramp Rate (A/min)") 0.5 ("Ramp Rate (A/min)") 1.0 ("Ramp Rate (A/min)") 2.0 ("Ramp Rate (A/min)") 0.5 ("Ramp Rate (A/min)")] -> w514
              frame "Up to 45 A at 2 A/m", Default {
              }
              frame "Up to 63 A at 1 A/m" {
              }
              frame "Up to 74.51 A at 0.5 A/m" {
                (unwired) 74.78 ("Target Current")
              }
              frame "Up to 74.47 A at 0.5 A/m" {
              }
              frame "Down to 74 A at 0.5 A/m" {
              }
              frame "Down to 63 A at 0.5 A/m" {
              }
              frame "Down to 45 A at 1 A/m" {
              }
              frame "Down to 0 A at 2 A/m" {
              }
              frame "Down to 0 A at 0.5 A/m" {
              }
            }
            n198 = property on="Target Current" class="DigNum (strict)"("Val(Sgnl)"=w512) -> ()  [unwired: 2 in, 2 out]
            n199 = local write "Ramp Rate (A/min)"(w514) -> ()
          }
        }
      }
      event "LHe_probe_mode": Value Change {
        n200 = event-data() -> ()  [unwired: 1 in, 6 out]
        n201 = call "AMI1700eth_set_meas_mode.vi"("int_samp"="LHe_probe_int_samp", "mode"="LHe_probe_mode", "error in"=w533, "conn_id_in"=w542) -> ("error out"=w534:errorcluster, "conn_id_out"=w535:refnum<k5>)  [unwired: 6 in]
        n202 = local read "Timer"() -> (w538:dbl)
      }
      event "recon_ami1700": Value Change {
        n203 = event-data() -> ()  [unwired: 1 in, 6 out]
        n204 = local read "AMI1700_address"() -> (w557:string)
        n205 = local read "AMI1700_port"() -> (w556:u16)
        n206 = call "AMI1700eth_close.vi"("error in"=w551, "conn_id"=w558) -> ("error out"=w555:errorcluster)  [unwired: 8 in, 1 out]
        n207 = call <vilib>:"Clear Errors.vi"("error in (no error)"=w555) -> ("error out"=w554:errorcluster)  [unwired: 5 in, 1 out]
        n208 = call "AMI1700eth_init.vi"("error in"=w554, "port"=w556, "address"=w557) -> ("error out"=w552:errorcluster, "conn_id"=w553:refnum<k5>)  [unwired: 6 in, 1 out]
      }
    }
    "Timer" <- w138
    n209 = call "MiPS_set.vi"("Target Current"=w124, "Ramp Rate (A/min)"="Ramp Rate (A/min)", "error in"=w160, "ISOBUS address"=w129, "ref_in"=w125) -> ("error out"=w149:errorcluster, "PSU Act Stat"=w123:T1, "PSU Stat"=→"PSU_Stat":T1, "ref_out"=w150:T6, "iPS_msg"=→"iPS_msg":string, "Status Hex value"=w89:i32)  [unwired: 1 in]
    "PSU_stat_hex" <- w89
    n210 = case shown="\"CLMP\"" w123 {
      tunnel: [TRUE FALSE FALSE TRUE] -> w155
      tunnel: [FALSE TRUE FALSE FALSE] -> w152
      tunnel: [FALSE FALSE TRUE FALSE] -> w153
      tunnel: [FALSE ("Blinking") FALSE ("Blinking") FALSE ("Blinking") TRUE ("Blinking")] -> w154
      tunnel: [TRUE FALSE FALSE TRUE] -> w118
      tunnel: [FALSE FALSE FALSE TRUE ("Blinking")] -> w91
      frame "HOLD", Default {
      }
      frame "RTOS" {
      }
      frame "RTOZ" {
      }
      frame "CLMP" {
      }
    }
    "Holdlight" <- w155
    "Setlight" <- w152
    "Zerolight" <- w153
    "clamped_light" <- w91
    n211 = And(x=w89, y=16) -> (x .and. y?=w87:i32)
    n212 = call "status_bool_to_color.vi"("status_bool_3"=w101, "status_bool_2"=w75, "status_bool_1"=w103) -> ("status_color"=w102:u32)  [unwired: 8 in]
    n213 = Not Equal To 0?(x=w87) -> (x != 0?=→"quenched_light":bool)
    n214 = global write "Magnet_PS_Global.vi" "MagPS_ST"(w102) -> ()
    n215 = property on="Holdlight" class="Bool (strict)"("Blinking"=w154) -> ()  [unwired: 2 in, 2 out]
    "big_message" <- "SWITCH HEATER CHANGING STATE, PLEASE WAIT" ("String")
    "Baselinetext" <- "BASELINE MODE" ("Baselinetext")
  }
  n216 = flat-sequence {
    tunnel: w15 -> [w572]
    tunnel: w14 -> [w571]
    tunnel: w10 -> [w570]
    tunnel: w9 -> [w569]
    tunnel: w6 -> [w568]
    tunnel: w4 -> [w565]
    tunnel: w2 -> [w564]
    frame #0 {
      w566 = 0.0 ("MagPS_LHe")
      n217 = call "Close.vi"("error in (no error)"=w571, "Mercury Reference"=w572) -> ("error out"=w559:errorcluster)  [unwired: 9 in]
      n218 = call "SR201_close.vi"("conn_id"=w568) -> ("error out"=w560:errorcluster)  [unwired: 9 in, 1 out]
      n219 = call "AMI1700eth_close.vi"("error in"=w569, "conn_id"=w570) -> ("error out"=w561:errorcluster)  [unwired: 8 in, 1 out]
      n220 = VISA Close(VISA resource name=w565, error in (no error)=w564) -> (error out=w563:errorcluster)
      n221 = call <vilib>:"Clear Errors.vi"("error in (no error)"=w559) -> ()  [unwired: 5 in, 2 out]
      n222 = call <vilib>:"Clear Errors.vi"("error in (no error)"=w560) -> ()  [unwired: 5 in, 2 out]
      n223 = call <vilib>:"Clear Errors.vi"("error in (no error)"=w561) -> ()  [unwired: 5 in, 2 out]
      n224 = global write "Magnet_PS_Global.vi" "MagPS_ST"(u32 0 ("MagPS_ST")) -> ()
      n225 = global write "Magnet_PS_Global.vi" "MagPS_LHe"(w566) -> ()
      n226 = global write "Magnet_PS_Global.vi" "MagPS_LN2"(w566) -> ()
      n227 = call <vilib>:"Clear Errors.vi"("error in (no error)"=w563) -> ()  [unwired: 5 in, 2 out]
      n228 = local write "curr_preset"(T2."None" ("curr_preset")) -> ()
    }
  }
